vi "LeCroy - Acquire Timed Sequence.vi"() -> ()   [LabVIEW 8.6]
doc: "This example configures the sequence acquisition mode, initiates the acquisition, waits for the acquisition to complete and reads all acquired segments. The segment data contain timestamping information.\n\nNote:\n\nSequence Acquisitions are not supported by WaveSurfer models."
panel:
  in  "Number of Segments (2)":u16
  in  "Source (0: Channel 1)":u16(ring) items=["Channel 1", "Channel 2", "Channel 3", "Channel 4", "Memory 1", "Memory 2", "Memory 3", "Memory 4", "Function 1", "Function 2", "Function 3", "Function 4", "Function 5", "Function 6", "Function 7", "Function 8"]
  out "Waveform Data":waveform(dbl)[](graph)
  in  "Timeout (10000 ms)":u32
  in  "VISA resource name":refnum<visa-resource-name>
  # "(c) 2008 NATIONAL INSTRUMENTS.  ALL RIGHTS RESERVED."
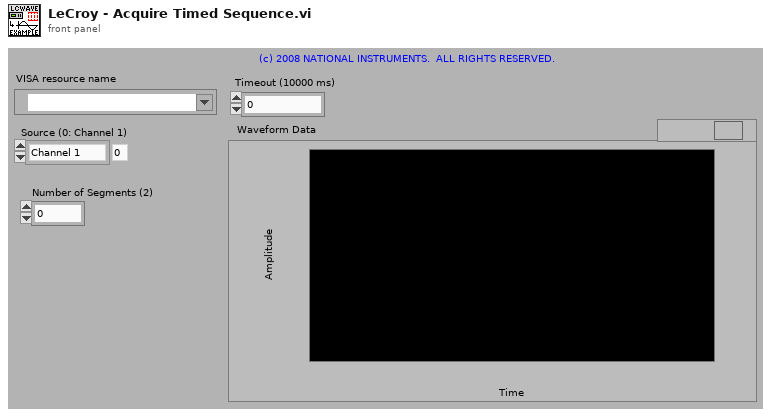
[diagram p1: front panel]
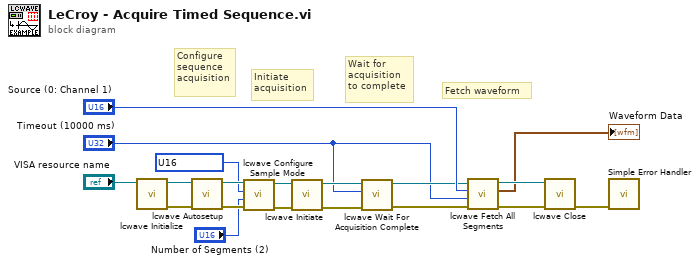
[diagram p0: block diagram]
diagram:
  w2 = u16 ? items=["RealTime", "RIS", "Sequence", "Roll", "WaveStream"] ("Sample Mode (0: RealTime)")
  # "Fetch waveform"
  # "Wait for \nacquisition\nto complete"
  # "Initiate\nacquisition"
  # "Configure sequence\nacquisition"
  n1 = call "lcwave Initialize.vi"("VISA resource name"="VISA resource name") -> ("error out"=w8:errorcluster, "VISA resource name out"=w9:refnum<visa-resource-name>)  [unwired: 9 in]
  n2 = call "lcwave Autosetup.vi"("error in (no error)"=w8, "VISA resource name"=w9) -> ("error out"=w5:errorcluster, "VISA resource name out"=w6:refnum<visa-resource-name>)  [unwired: 8 in]
  n3 = call "lcwave Configure Sample Mode.vi"("error in (no error)"=w5, "Number of Segments (2)"="Number of Segments (2)", "Sample Mode (0: RealTime)"=w2, "VISA resource name"=w6) -> ("error out"=w4:errorcluster, "VISA resource name out"=w3:refnum<visa-resource-name>)  [unwired: 6 in]
  n4 = call "lcwave Initiate.vi"("error in (no error)"=w4, "VISA resource name"=w3) -> ("error out"=w10:errorcluster, "VISA resource name out"=w13:refnum<visa-resource-name>)  [unwired: 8 in]
  n5 = call "lcwave Wait For Acquisition Complete.vi"("error in (no error)"=w10, "Timeout (10000 ms)"="Timeout (10000 ms)", "VISA resource name"=w13) -> ("error out"=w11:errorcluster, "VISA resource name out"=w12:refnum<visa-resource-name>)  [unwired: 6 in, 1 out]
  n6 = call "lcwave Fetch All Segments.vi"("error in (no error)"=w11, "Timeout (10000 ms)"="Timeout (10000 ms)", "Source (0: Channel 1)"="Source (0: Channel 1)", "VISA resource name"=w12) -> ("error out"=w17:errorcluster, "Array"=→"Waveform Data":waveform(dbl)[], "VISA resource name out"=w18:refnum<visa-resource-name>)  [unwired: 5 in]
  n7 = call "lcwave Close.vi"("error in (no error)"=w17, "VISA resource name"=w18) -> ("error out"=w19:errorcluster)  [unwired: 9 in]
  n8 = call <vilib>:"Simple Error Handler.vi"("error in (no error)"=w19) -> ()  [unwired: 4 in, 5 out]
